vi "absCalibrate.vi"(5 "Calibrant xsec 532 (cm^2/molec)":dbl=1.5e-19, 6 "[Calibrant] (molec/cc)":dbl=250000000000000.0, 7 "Calibrant xsec 660 (cm^2/molec) 2":dbl, 8 "calibrant flows (sccm)":dbl[](array[numeric]), 9 "dilution flows (sccm)":dbl[](array[numeric]), 10 "532 Intensities":cluster{"532 I":dbl[], "532 I0":dbl[]}, 11 "660 Intensities":cluster{"660 I":dbl[], "660 I0":dbl[]}) -> (2 "660 Calibration":T1, 3 "532 Calibration":T1 {"?"."abs (1/cm)" format="%#_4p"})   [LabVIEW 2011]
uses:
  <vilib>/Analysis/NI_AALPro.lvlib
  <vilib>/gmath/NI_Gmath.lvlib
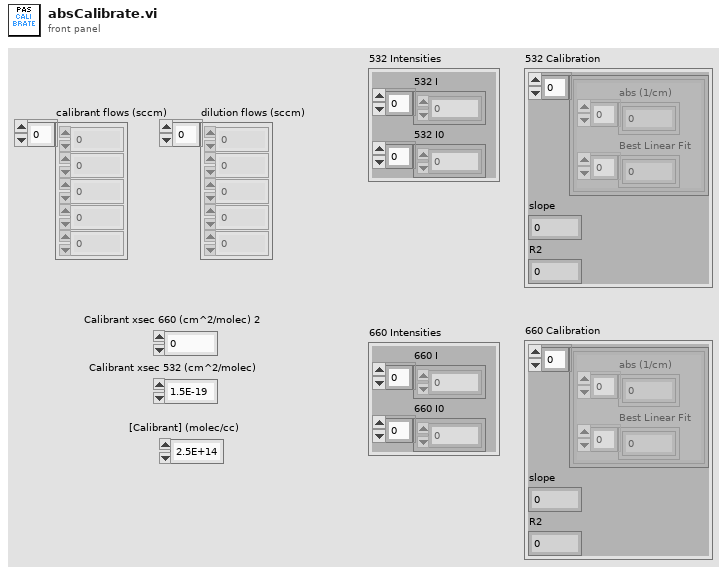
[diagram p1: front panel]
types:
  T1 = cluster{cluster{"abs (1/cm)":dbl[], "Best Linear Fit":dbl[]}[], "slope":dbl, "R2":dbl}
  T2 = cluster{"slope min":dbl, "slope max":dbl, "intercept min":dbl, "intercept max":dbl}
  T3 = cluster{"Abs (1/Mm)":dbl[], "Best Linear Fit":dbl[]}
  T4 = cluster{"Abs (1/Mm)":dbl[], "Best Linear Fit":dbl[]}[]
  T5 = cluster{cluster{"Abs (1/Mm)":dbl[], "Best Linear Fit":dbl[]}[], "slope":dbl, "correlation coefficient r":dbl}
  T6 = cluster{cluster{"Abs (1/Mm)":dbl[], "Best Linear Fit":dbl[]}[], "slope":dbl, "r^2":dbl}
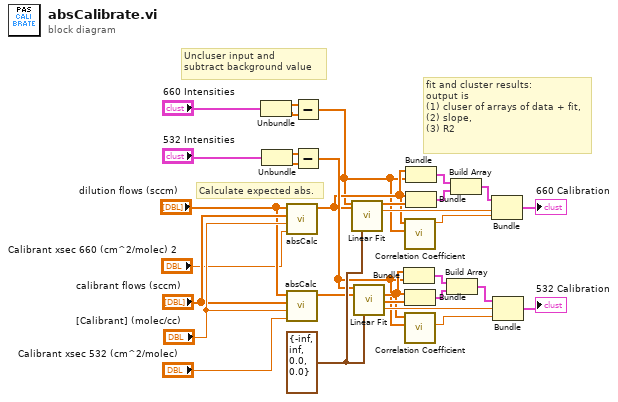
[diagram p0: block diagram]
diagram:
  w29 = T2 {"slope min"=-inf, "slope max"=inf, "intercept min"=0.0, "intercept max"=0.0} ("parameter bounds")
  # "Calculate expected abs."
  # "fit and cluster results:\noutput is \n(1) cluser of arrays of data + fit,\n(2) slope,\n(3) R2"
  # "Uncluser input and \nsubtract background value"
  n1 = Unbundle("660 Intensities") -> ("660 I"=w20:dbl[], "660 I0"=w19:dbl[])
  n2 = Unbundle("532 Intensities") -> ("532 I"=w18:dbl[], "532 I0"=w17:dbl[])
  n3 = call "absCalc.vi"("Calibrant xssc (cm^2/molec)"="Calibrant xsec 660 (cm^2/molec) 2", "[Calibrant] (molec/cc)"="[Calibrant] (molec/cc)", "calibrant flows (sccm)"="calibrant flows (sccm)", "dilution flows (sccm)"="dilution flows (sccm)") -> ("Abs (1/Mm)"=w2:dbl[])  [unwired: 7 in]
  n4 = call "absCalc.vi"("Calibrant xssc (cm^2/molec)"="Calibrant xsec 532 (cm^2/molec)", "[Calibrant] (molec/cc)"="[Calibrant] (molec/cc)", "calibrant flows (sccm)"="calibrant flows (sccm)", "dilution flows (sccm)"="dilution flows (sccm)") -> ("Abs (1/Mm)"=w6:dbl[])  [unwired: 7 in]
  n5 = Subtract(x=w20, y=w19) -> (x-y=w1:dbl[])
  n6 = Subtract(x=w18, y=w17) -> (x-y=w5:dbl[])
  n7 = call <vilib>:"Linear Fit.vi"("Y"=w1, "X"=w2, "parameter bounds"=w29) -> ("Best Linear Fit"=w9:dbl[], "slope"=w30:dbl)  [unwired: 8 in, 3 out]
  n8 = call <vilib>:"Linear Fit.vi"("Y"=w5, "X"=w6, "parameter bounds"=w29) -> ("Best Linear Fit"=w13:dbl[], "slope"=w28:dbl)  [unwired: 8 in, 3 out]
  n9 = Bundle("Abs (1/Mm)"=w6, w5) -> (w12:cluster{"Abs (1/Mm)":dbl[], dbl[]})  [unwired: 1 in]
  n10 = call <vilib>:"Correlation Coefficient.vi"("Y"=w1, "X"=w2) -> ("correlation coefficient r"=w3:dbl)  [unwired: 8 in, 1 out]
  n11 = Bundle("Abs (1/Mm)"=w6, "Best Linear Fit"=w13) -> (w11:T3)  [unwired: 1 in]
  n12 = call <vilib>:"Correlation Coefficient.vi"("Y"=w5, "X"=w6) -> ("r^2"=w4:dbl)  [unwired: 8 in, 1 out]
  n13 = Bundle("Abs (1/Mm)"=w2, w1) -> (w16:cluster{"Abs (1/Mm)":dbl[], dbl[]})  [unwired: 1 in]
  n14 = Bundle("Abs (1/Mm)"=w2, "Best Linear Fit"=w9) -> (w15:T3)  [unwired: 1 in]
  n15 = Build Array(w12, w11) -> (w10:T4)
  n16 = Build Array(w16, w15) -> (w14:T4)
  n17 = Bundle(w14, "slope"=w30, "correlation coefficient r"=w3) -> (→"660 Calibration":T5)  [unwired: 1 in]
  n18 = Bundle(w10, "slope"=w28, "r^2"=w4) -> (→"532 Calibration":T6)  [unwired: 1 in]
